vi "未命名 1.vi"() -> ()   [LabVIEW 2010]
uses:
  <vilib>/AddOns/Modulation/Analog/controls/Complex Data Waveform.ctl
  <vilib>/addons/Modulation/Digital/General/MT Generate Bits (Galois, PN Order).vi
  <vilib>/addons/Modulation/Digital/Impairments/Fading Profiles/MT Rician Fading Profile (Jakes).vi
  <vilib>/Analysis/2dsp.llb/Complex FFT.vi
  <vilib>/AddOns/Modulation/Digital/General/MT Apply Pulse Shaping Filter (Generic).vi
  <vilib>/AddOns/Modulation/Digital/General/MT Apply Matched Filter (Generic).vi
  <vilib>/addons/Adaptive Filters/Create/AFT Create FIR LMS (Complex).vi
  <vilib>/addons/Adaptive Filters/Processing/AFT Filter Signal and Update Coefficients (Complex, Array).vi
  <vilib>/imath/engines/lvmath2/RunTimeEngine/ErrorHandling/NIMS_Finalize Error.vi
  <vilib>/imath/engines/lvmath2/RunTimeEngine/Managers/WorkSpace/UID Generator.vi
  <vilib>/imath/engines/lvmath2/RunTimeEngine/Managers/SymbolTable/Clear UID.vi
  <vilib>/imath/engines/lvmath2/RunTimeEngine/NodeEndStatement/NIMS_NodeEndStatement_Output.vi
  <instcachedir>/0/NIMS_NodeEndStatement_Output_53EC0D466D134D7ABD903AC30B43404B.lvgen/NIMS_NodeEndStatement_Output_53EC0D466D134D7ABD903AC30B43404B_000.vi
  <vilib>/imath/engines/lvmath2/RunTimeEngine/BuiltInFunctions/length/NIMS_length(GV).vi
  <instcachedir>/0/NIMS_length(GV)_08A3D13377FD4E4B96F5795FBF3698FA.lvgen/NIMS_length(GV)_08A3D13377FD4E4B96F5795FBF3698FA_002.vi
  <vilib>/imath/engines/lvmath2/RunTimeEngine/RunTimeType/NIMS_RunTimeType_From StrictType (excl LVString).vi
  <vilib>/imath/engines/lvmath2/RunTimeEngine/LocalVariableDefStatement/MC_LocalVariableDefStatement_Display.vi
  <vilib>/imath/engines/lvmath2/RunTimeEngine/BuiltInFunctions/zeros/NIMS_V=zeros(I32,I32).vi
  <vilib>/imathl/engines/lvmath/Functions/Error Handling/Create Error.vi
  <vilib>/imath/engines/lvmath2/RunTimeEngine/RangeToken/NIMS_Range_R2 - Integer.vi
  <instcachedir>/0/NIMS_Range_R2 - Integer_217CA55F27D14E80B3D190635C7B3F47.lvgen/NIMS_Range_R2 - Integer_217CA55F27D14E80B3D190635C7B3F47_000.vi
  <vilib>/imath/engines/lvmath2/RunTimeEngine/CommandStatement/MC_CommandStatement_break.vi
  <vilib>/imath/engines/lvmath2/RunTimeEngine/VariableToken/Read/NIMS_Get Elements - RV(_) - Check.vi
  <instcachedir>/0/NIMS_Get Elements - RV(_) - Check_1F6F8656162345078B1D4DC9877DFAE9.lvgen/NIMS_Get Elements - RV(_) - Check_1F6F8656162345078B1D4DC9877DFAE9_004.vi
  <vilib>/imath/engines/lvmath2/RunTimeEngine/ReplaceToken/NIMS_Replace - Check Linear.vi
  <instcachedir>/0/NIMS_Replace - Check Linear_662D5651E4E34E0584DA82A256193A4C.lvgen/NIMS_Replace - Check Linear_662D5651E4E34E0584DA82A256193A4C_002.vi
  <vilib>/imath/engines/lvmath2/RunTimeEngine/ReplaceToken/NIMS_Replace - Size Check _(_)=S.vi
  <instcachedir>/0/NIMS_Replace - Size Check _(_)=S_6CAC13ACC74349C582FDAB09BCDAB70F.lvgen/NIMS_Replace - Size Check _(_)=S_6CAC13ACC74349C582FDAB09BCDAB70F_001.vi
  <vilib>/imath/engines/lvmath2/RunTimeEngine/ReplaceToken/NIMS_Replace - V(S)=S.vi
  <instcachedir>/0/NIMS_Replace - V(S)=S_78FDB6CCD265407D8926E4CF958018EB.lvgen/NIMS_Replace - V(S)=S_78FDB6CCD265407D8926E4CF958018EB_001.vi
  <instcachedir>/0/NIMS_length(GV)_08A3D13377FD4E4B96F5795FBF3698FA.lvgen/NIMS_length(GV)_08A3D13377FD4E4B96F5795FBF3698FA_001.vi
  <vilib>/imath/engines/lvmath2/RunTimeEngine/RangeToken/NIMS_Range_R2 - Float.vi
  <instcachedir>/0/NIMS_Range_R2 - Float_B141A161314947C2A0872DED502D7279.lvgen/NIMS_Range_R2 - Float_B141A161314947C2A0872DED502D7279_000.vi
  <vilib>/imath/engines/lvmath2/RunTimeEngine/VariableToken/Read/NIMS_Get Elements - RV(_) - Check(_).vi
  <instcachedir>/0/NIMS_Get Elements - RV(_) - Check(_)_260A45C9C4AF472A8F32F86A1BEF7DEE.lvgen/NIMS_Get Elements - RV(_) - Check(_)_260A45C9C4AF472A8F32F86A1BEF7DEE_002.vi
  <vilib>/imath/engines/lvmath2/RunTimeEngine/ReplaceToken/NIMS_Replace - Check(_) Linear.vi
  <instcachedir>/0/NIMS_Replace - Check(_) Linear_D531E313C4004E3DB8F0EA3CE86AE758.lvgen/NIMS_Replace - Check(_) Linear_D531E313C4004E3DB8F0EA3CE86AE758_008.vi
  <vilib>/Analysis/2dsp.llb/Inverse Complex FFT.vi
  <vilib>/addons/Modulation/niDMT.lvlib
  <vilib>/Analysis/NI_AALPro.lvlib
  <vilib>/addons/Modulation/niAMT.lvlib
  <vilib>/addons/Adaptive Filters/NI_AdaptiveFilter.lvlib
  <vilib>/imath/engines/lvmath2/RunTimeEngine/Managers/SymbolTable/NIMS_WorkSpace.lvlib
  <vilib>/addons/Modulation/Digital/Impairments/MT Apply Flat Fading Profile.vi
panel:
  out "大小 3":i32
  out "Y 4":dbl[](graph)
  out "大小 2":i32
  out "大小":i32
  out "Y 3":dbl[](graph)
  out "Y 2":dbl[](graph)
  out "Y":dbl[](graph)
  out "波形图":dbl[](graph)
  out "matched filter coefficients":dbl[](graph)
  out "pulse shaping filter coefficients":dbl[](graph)
  out "TX Constellation":T1(graph)
  out "constellation graph":T2(graph)
  out "X":dbl[](graph)
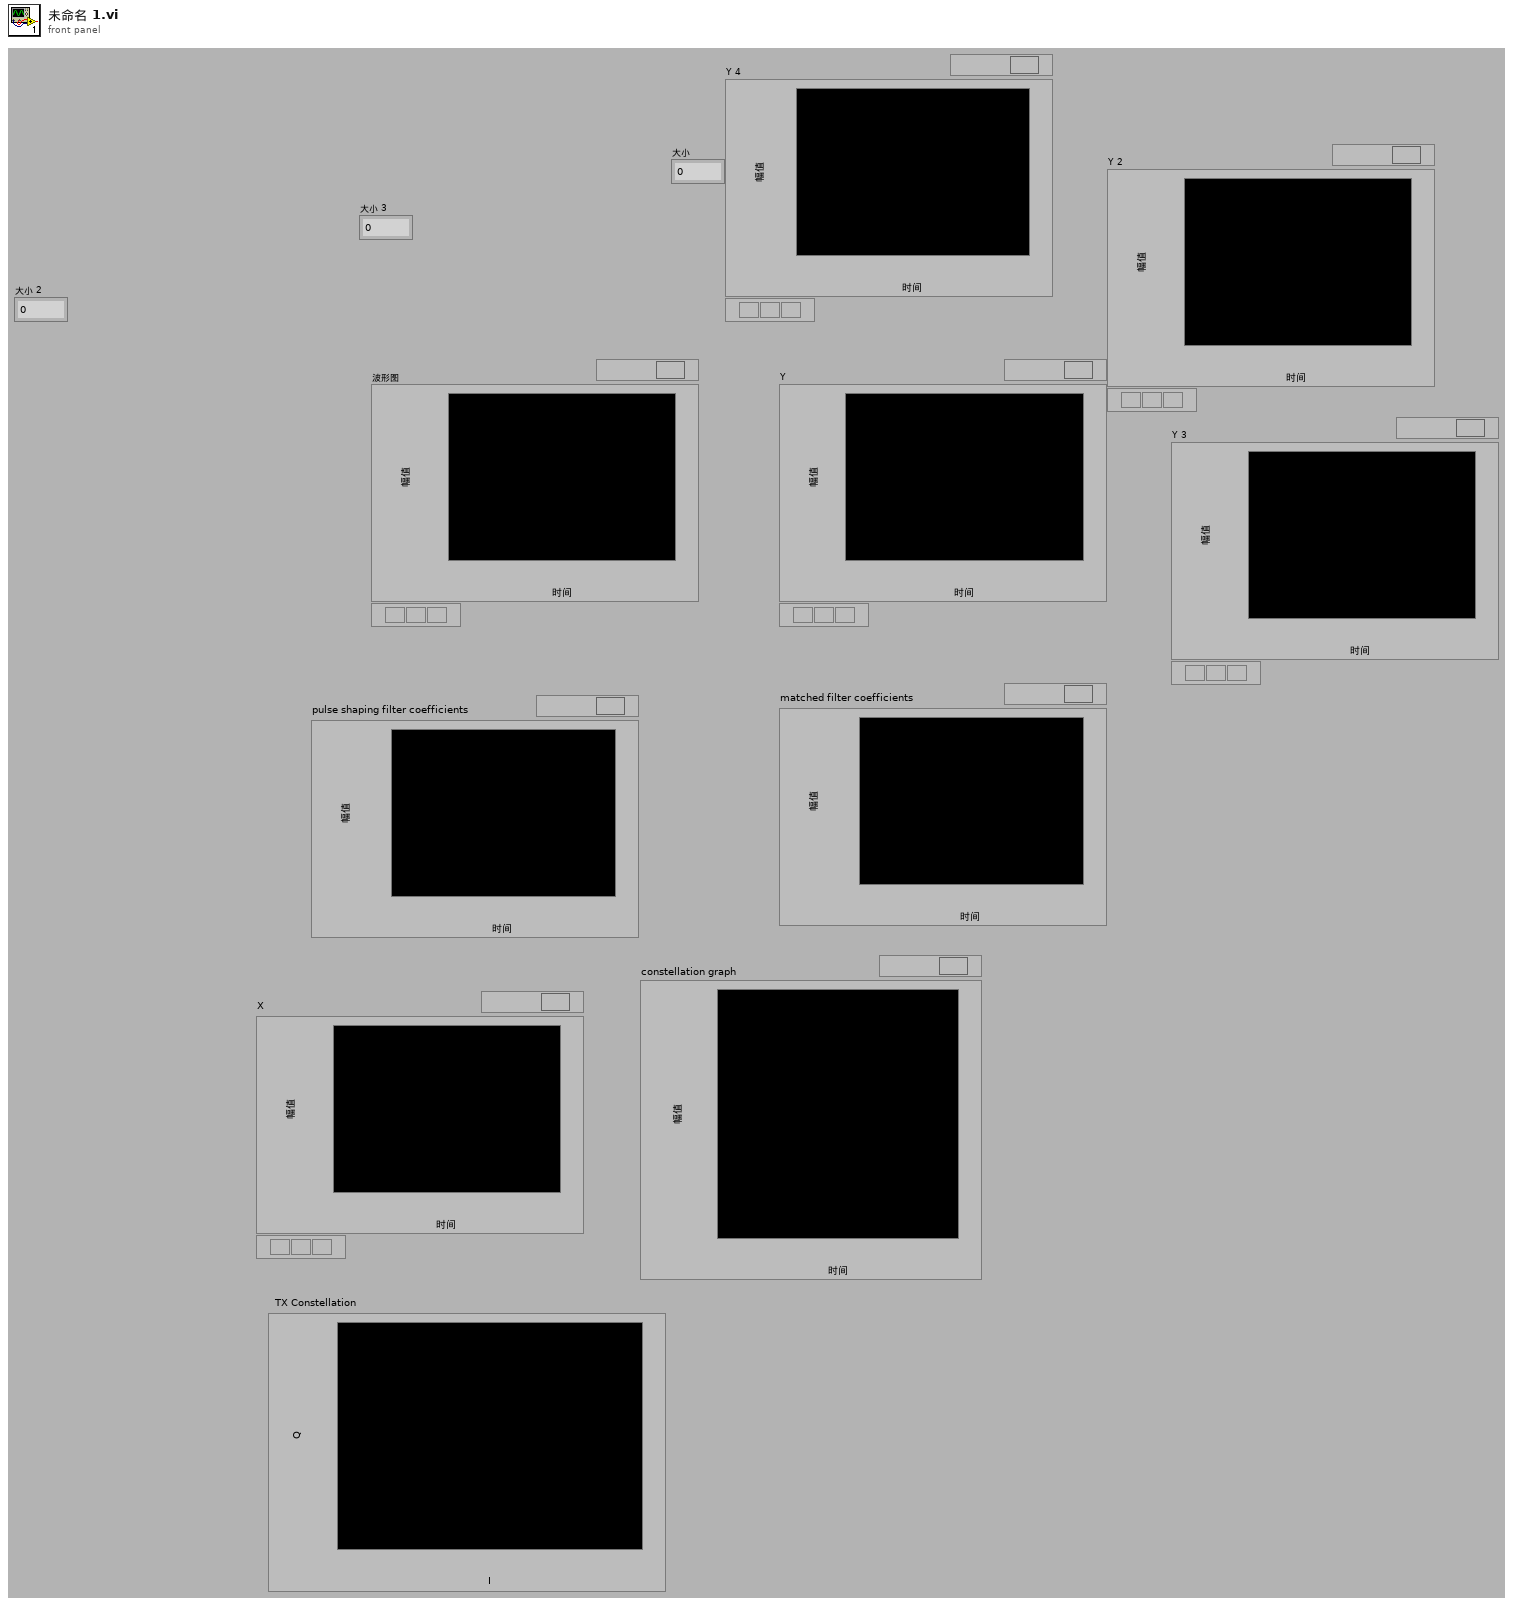
[diagram p1: front panel]
types:
  T1 = cluster{"Decimated Array":dbl[], "Decimated Array":dbl[]}[]
  T2 = cluster{"constellation":dbl[], "oversampled data":dbl[]}[]
  T3 = enum16{"FSK", "PSK", "QAM", "MSK", "PAM", "ASK", "CPM"}
  T4 = enum16{"none", "Raised Cosine", "Root Raised Cos", "Gaussian"}
  T5 = typedef "niAMT.lvlib/Complex Data Waveform.ctl" = cluster{"t0":dbl, "dt":dbl, "Y":cdb[]}
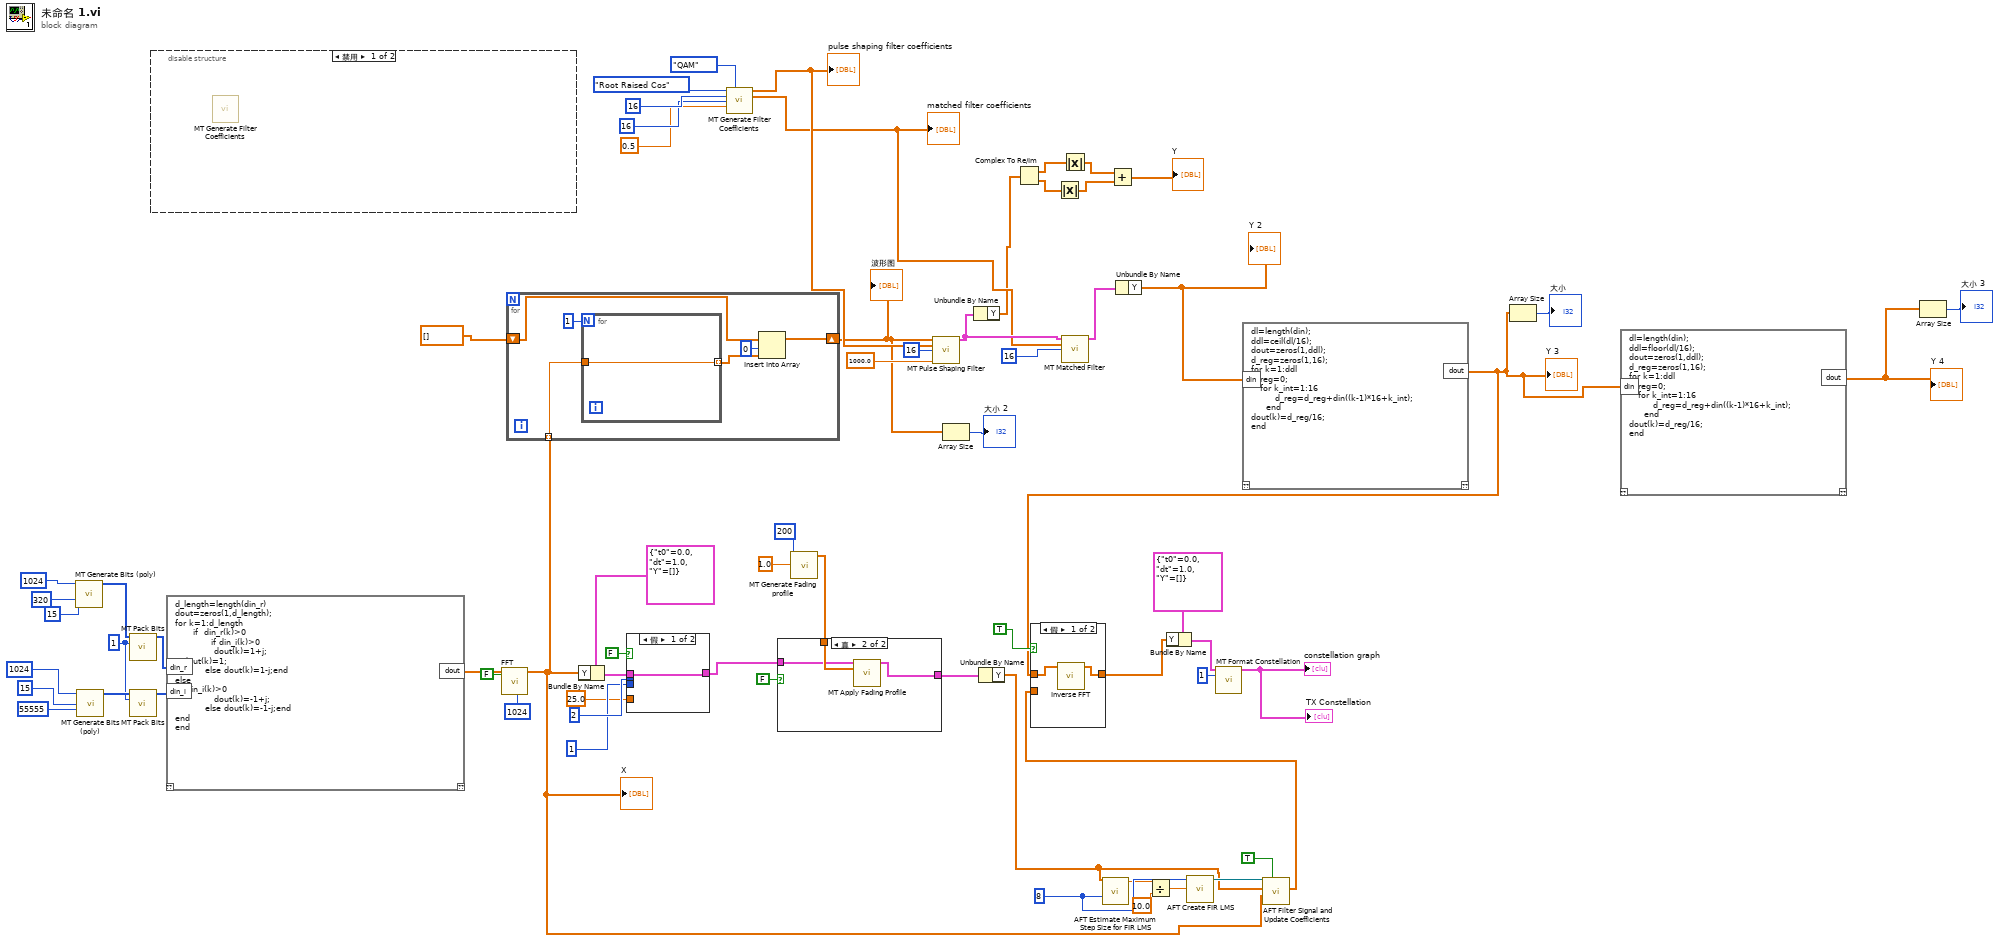
[diagram p0: block diagram]
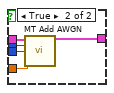
[diagram p4: hidden frame]
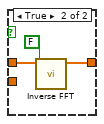
[diagram p5: hidden frame]
diagram:
  w45 = 8 ("filter length")
  w60 = 1 ("bits per integer")
  n1 = call-poly <vilib>:"MT Generate Bits (poly).vi"("total bits (128)"=1024, "PN sequence order (9)"=15, "seed in (0xD6BF7DF2)"=320) -> ("output bit stream"=w66:i8[])  [unwired: 10 in, 2 out]
  n2 = call-poly <vilib>:"MT Generate Bits (poly).vi"("total bits (128)"=1024, "PN sequence order (9)"=15, "seed in (0xD6BF7DF2)"=55555) -> ("output bit stream"=w62:i8[])  [unwired: 10 in, 2 out]
  n3 = call <vilib>:"MT Pack Bits.vi"("input bit stream"=w66, "bits per integer"=w60) -> ("output integers"=w57:i32[])  [unwired: 12 in, 1 out]
  n4 = call <vilib>:"MT Pack Bits.vi"("input bit stream"=w62, "bits per integer"=w60) -> ("output integers"=w58:i32[])  [unwired: 12 in, 1 out]
  n5 = disable-structure shown="禁用" {
    frame Disabled {
      n6 = call <vilib>:"MT Generate Filter Coefficients.vi"() -> ()  [unwired: 13 in, 3 out]
    }
    frame Enabled {
    }
  }
  n7 = mathscript code="d_length=length(din_r)\ndout=zeros(1,d_length);\nfor k=1:d_length\n      if  din_r(k)>0\n            if din_i(k)>0\n             dout(k)=1+j;\n%dout(k)=1;\n          else dout(k)=1-j;end\nelse   \n if din_i(k)>0\n             dout(k)=-1+j;\n          else dout(k)=-1-j;end\nend\nend"("din_r"=w57, "din_i"=w58) -> ("dout"=w41:cdb[])  [unwired: 1 in, 1 out]
  n8 = call-poly <vilib>:"FFT.vi"("FFT size"=1024, "shift?"=FALSE, "X"=w41) -> ("FFT {X}"=w22:cdb[])  [unwired: 7 in, 1 out]
  "X" <- w22
  n9 = for {
    tunnel: w22 -> [w73] mode=indexing
    shift-right: [w68] -> w10
    shift-left: cdb[] [] ("数组") -> [w71]
    n10 = for {
      N: 1 -> [_]
      tunnel: w73 -> [w74]
      tunnel: [w74] -> w70 mode=indexing
    }
    n11 = Insert Into Array(array=w71, index=0 ("索引"), new element=w70) -> (w68:cdb[])
  }
  "波形图" <- w10
  n12 = Bundle By Name(cluster=T5 {"t0"=0.0, "dt"=1.0, "Y"=[]} ("input complex waveform"), "Y"=w22) -> (w54:T5)
  n13 = case shown="假" FALSE {
    tunnel: 2 ("samples per symbol (16)") -> [_ w80]
    tunnel: w54 -> [w75 w79]
    tunnel: 1 ("bits per symbol (1)") -> [_ w78]
    tunnel: 25.0 ("Eb/N0 (10 dB)") -> [_ w77]
    tunnel: [w75 w76] -> w35
    frame False {
    }
    frame True {
      n14 = call <vilib>:"MT Add AWGN.vi"("input complex waveform"=w79, "samples per symbol (16)"=w80, "bits per symbol (1)"=w78, "Eb/N0 (10 dB)"=w77) -> ("output complex waveform"=w76:T5)  [unwired: 9 in, 2 out]
    }
  }
  n15 = call <vilib>:"MT Generate Filter Coefficients.vi"("pulse shaping filter (none)"=T4."Root Raised Cos", "modulation type"=T3."QAM", "pulse shaping samples per symbol (16)"=16, "matched samples per symbol (16)"=16, "filter parameter"=0.5) -> ("pulse shaping filter coefficients"=w20:dbl[], "matched filter coefficients"=w16:dbl[])  [unwired: 8 in, 1 out]
  "pulse shaping filter coefficients" <- w20
  "matched filter coefficients" <- w16
  n16 = call-poly <vilib>:"MT Generate Fading profile.vi"("profile length (samples)"=200, "sampling frequency (Hz)"=1.0) -> ("fading profile"=w36:cdb[])  [unwired: 11 in, 2 out]
  n17 = case shown="真" FALSE {
    tunnel: w36 -> [_ w84]
    tunnel: w35 -> [w81 w83]
    tunnel: [w81 w82] -> w34
    frame False {
    }
    frame True {
      n18 = call-poly <vilib>:"MT Apply Fading Profile.vi"("input complex waveform"=w83, "fading profile"=w84) -> ("output complex waveform"=w82:T5)  [unwired: 12 in, 1 out]
    }
  }
  n19 = call-poly <vilib>:"MT Pulse Shaping Filter.vi"("symbols"=w10, "pulse shaping filter coefficients"=w20, "samples per symbol (16)"=16, "symbol rate (Hz)"=1000.0) -> ("output complex waveform"=w17:T5)  [unwired: 10 in, 1 out]
  n20 = Array Size(array=w10) -> (size(s)=→"大小 2":i32)
  n21 = Unbundle By Name(w17) -> ("Y"=w7:cdb[])
  n22 = Unbundle By Name(w34) -> ("Y"=w32:cdb[])
  n23 = Complex To Re/Im(x + iy=w7) -> (x=w6:dbl[], y=w5:dbl[])
  n24 = Absolute Value(x=w5) -> (abs(x)=w3:dbl[])
  n25 = Absolute Value(x=w6) -> (abs(x)=w4:dbl[])
  n26 = call-poly <vilib>:"MT Matched Filter.vi"("input complex waveform"=w17, "matched filter coefficients"=w16, "samples per symbol (16)"=16) -> ("output complex waveform"=w14:T5)  [unwired: 11 in, 1 out]
  n27 = call <vilib>:"AFT Estimate Maximum Step Size for FIR LMS.vi"("filter length"=w45, "x(n)"=w32) -> ("maximum step size"=w30:dbl)  [unwired: 8 in, 1 out]
  n28 = Add(x=w4, y=w3) -> (x+y=→"Y":dbl[])
  n29 = Unbundle By Name(w14) -> ("Y"=w12:cdb[])
  "Y 2" <- w12
  n30 = Divide(x=w30, y=10.0) -> (x/y=w31:dbl)
  n31 = call-poly <vilib>:"AFT Create FIR LMS.vi"("step size"=w31, "filter length"=w45) -> ("adaptive filter out"=w44:refnum<k20>)  [unwired: 8 in, 1 out]
  n32 = mathscript code="dl=length(din);\nddl=ceil(dl/16);\ndout=zeros(1,ddl);\nd_reg=zeros(1,16);\nfor k=1:ddl\nd_reg=0;\n   for k_int=1:16\n        d_reg=d_reg+din((k-1)*16+k_int);\n     end\ndout(k)=d_reg/16;\nend"("din"=w12) -> ("dout"=w2:cdb[])  [unwired: 1 in, 1 out]
  "Y 3" <- w2
  n33 = call-poly <vilib>:"AFT Filter Signal and Update Coefficients.vi"("reset? (F)"=TRUE, "d(n)"=w22, "x(n)"=w32, "adaptive filter in"=w44) -> ("y(n)"=w40:cdb[])  [unwired: 4 in, 3 out]
  n34 = case shown="假" TRUE {
    tunnel: [w86 w88] -> w42
    tunnel: w2 -> [w85 w87]
    tunnel: w40 -> [_ _]
    frame False {
      n35 = call-poly <vilib>:"Inverse FFT.vi"("FFT {X}"=w85) -> ("X"=w86:cdb[])  [unwired: 9 in, 1 out]
    }
    frame True {
      n36 = call-poly <vilib>:"Inverse FFT.vi"("shift?"=FALSE, "FFT {X}"=w87) -> ("X"=w88:cdb[])  [unwired: 8 in, 1 out]
    }
  }
  n37 = Bundle By Name(cluster=T5 {"t0"=0.0, "dt"=1.0, "Y"=[]} ("waveform"), "Y"=w42) -> (w49:T5)
  n38 = call <vilib>:"MT Format Constellation.vi"("waveform"=w49, "samples per symbol"=1) -> ("constellation graph"=→"constellation graph" →"TX Constellation":T2)  [unwired: 12 in, 1 out]
  n39 = Array Size(array=w2) -> (size(s)=→"大小":i32)
  n40 = mathscript code="dl=length(din);\nddl=floor(dl/16);\ndout=zeros(1,ddl);\nd_reg=zeros(1,16);\nfor k=1:ddl\nd_reg=0;\n   for k_int=1:16\n        d_reg=d_reg+din((k-1)*16+k_int);\n     end\ndout(k)=d_reg/16;\nend"("din"=w2) -> ("dout"=w8:cdb[])  [unwired: 1 in, 1 out]
  "Y 4" <- w8
  n41 = Array Size(array=w8) -> (size(s)=→"大小 3":i32)
